vi "LVOOP_WriteLogFile.vi"(8 "error in (no error)":errorcluster caption="错误输入（无错误）", 11 "RunningLog 输入":refnum<class "RunningLog.lvclass">) -> (0 "error out":errorcluster caption="错误输出", 3 "RunningLog 输出":refnum<class "RunningLog.lvclass">)   [LabVIEW 2018, in "RunningLog.lvclass"]
uses:
  RunningLog.lvclass
  RunningLog.lvclass/RunningLog.ctl
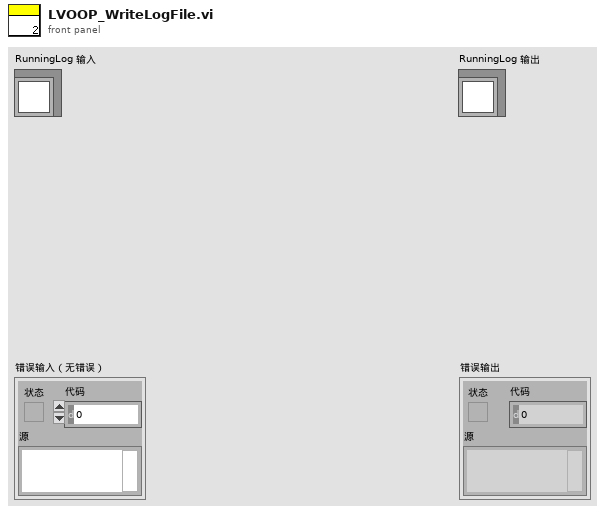
[diagram p1: front panel]
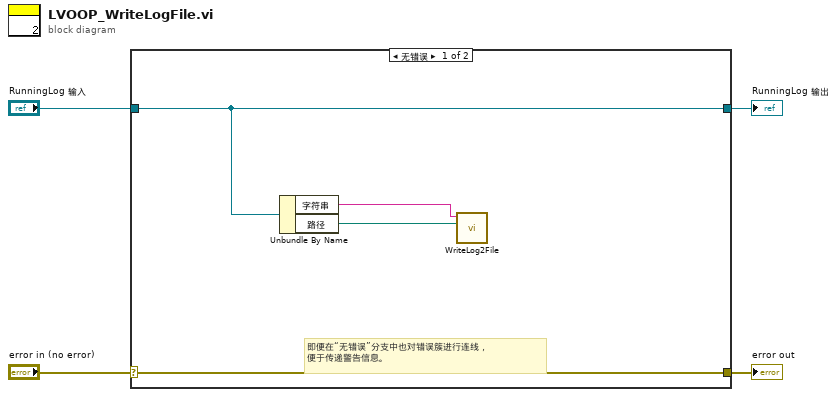
[diagram p0: block diagram]
diagram:
  n1 = case shown="无错误" "error in (no error)" {
    selector: "error in (no error)" -> [w8 w10]
    tunnel: [w8 w10] -> w3
    tunnel: [w5 w9] -> w1
    tunnel: "RunningLog 输入" -> [w5 w9]
    frame No Error {
      # "即便在“无错误”分支中也对错误簇进行连线，\n便于传递警告信息。"
      n2 = Unbundle By Name(w5) -> ("字符串"=w6:string, "路径"=w7:path)
      n3 = call "WriteLog2File.vi"("文件路径（使用对话框）"=w7, "文本"=w6) -> ()  [unwired: 9 in, 1 out]
    }
    frame Error {
    }
  }
  "error out" <- w3
  "RunningLog 输出" <- w1
